vi "autogen action.vi"(8 "error in":errorcluster, 9 "user event":T1, 10 "engine configuration in":refnum<class "engine configuration.lvclass">, 11 "UI Reference configuration in":refnum<class "UI Reference configuration.lvclass">=refnum) -> (0 "error out":errorcluster, 2 "engine configuration out":refnum<class "engine configuration.lvclass">, 3 "UI Reference configuration out":refnum<class "UI Reference configuration.lvclass">)   [LabVIEW 2014, in "UI Reference editor node.lvclass"]
uses:
  UI Reference editor node.lvclass
  <vilib>/NI/Configuration Framework/Controls/EventCluster.ctl
  <vilib>/NI/Configuration Framework/NISE_CEF_TreeControl.lvlib
  <vilib>/NI/Module Execution Interface/Engine Configuration/engine configuration.lvclass
  <vilib>/NI/Configuration Framework/serializable configuration/NISE_CEF_serializable configuration.lvclass
  module/configuration/UI Reference configuration.lvclass
  <vilib>/NI/Configuration Framework/Node/UserEventRef.ctl
  <vilib>/NI/Configuration Framework/Node/NISE_CEF_Node.lvclass
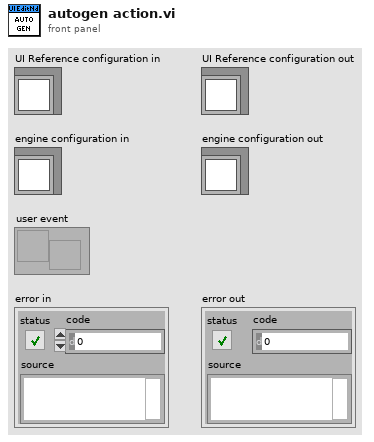
[diagram p1: front panel]
types:
  T1 = typedef "NISE_CEF_Node.lvclass/UserEventRef.ctl" = refnum<user-event>
  T2 = typedef "NISE_CEF_TreeControl.lvlib/EventCluster.ctl" = cluster{"command":string, "data":string}
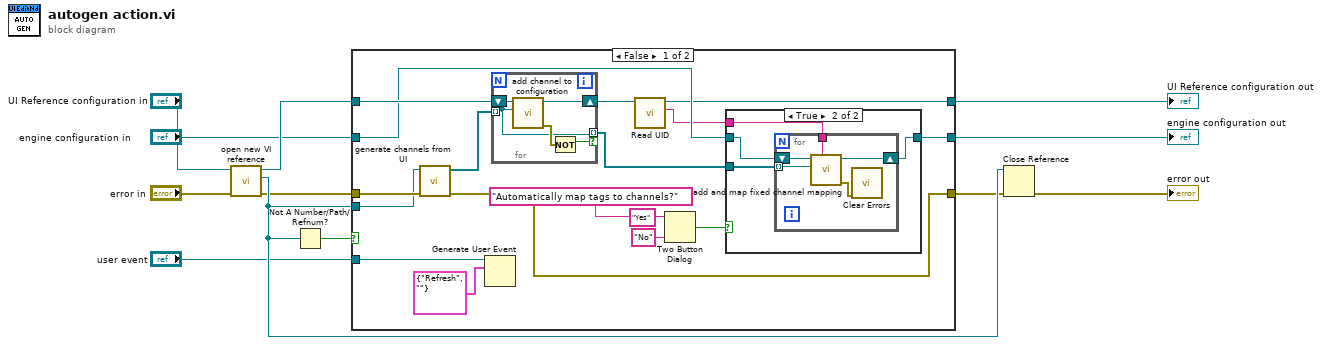
[diagram p0: block diagram]
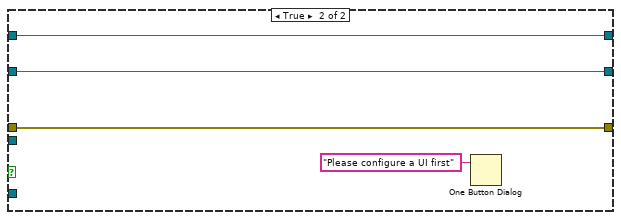
[diagram p3: hidden frame]
diagram:
  n1 = call "open new VI reference.vi"("error in"="error in", "UI Reference configuration in"="UI Reference configuration in") -> ("error out"=w7:errorcluster, "VI Refnum"=w9:refnum<vi>, "UI Reference configuration out"=w6:refnum<class "UI Reference configuration.lvclass">)  [unwired: 7 in]
  n2 = Not A Number/Path/Refnum?(number/path/refnum=w9) -> (NaN/Path/Refnum?=w1:bool)
  n3 = case shown="False" w1 {
    tunnel: w7 -> [w29 w46]
    tunnel: w6 -> [w27 w47]
    tunnel: [w20 w48] -> w11
    tunnel: "engine configuration in" -> [w21 w48]
    tunnel: [w14 w47] -> w12
    tunnel: [w18 w46] -> w3
    tunnel: w9 -> [w28 _]
    tunnel: "user event" -> [w16 _]
    frame False {
      n4 = call "generate channels from UI.vi"("error in"=w29, "VI Refnum"=w28) -> ("error out"=w18:errorcluster, "channels"=w26:refnum<class "TBM channel.lvclass">[])  [unwired: 8 in]
      n5 = Generate User Event(user event=w16, event data cluster=T2 {"command"="Refresh", "data"=""} ("event data")) -> ()  [unwired: 2 in, 2 out]
      n6 = for {
        tunnel: w26 -> [w41] mode=indexing
        shift-right: [w43] -> w22
        shift-left: w27 -> [w44]
        tunnel: [w41] -> w19 mode=indexing if=w40
        n7 = call "add channel to configuration.vi"("channel"=w41, "UI Reference configuration in"=w44) -> ("error out"=w42:errorcluster, "UI Reference configuration out"=w43:refnum<class "UI Reference configuration.lvclass">)  [unwired: 8 in]
        n8 = Not(x=w42) -> (.not. x?=w40:bool)
      }
      n9 = call <vilib>:"Read UID.vi"("configuration in"=w22) -> ("instance id"=w13:string, "configuration out"=w14:refnum<class "NISE_CEF_serializable configuration.lvclass">)  [unwired: 8 in, 1 out]
      n10 = Two Button Dialog(message="Automatically map tags to channels?", 1:"No" ("F button name (\"Cancel\")"), 2:"Yes" ("T button name (\"OK\")")) -> (T button?=w23:bool)
      n11 = case shown="True" w23 {
        tunnel: w21 -> [w30 w34]
        tunnel: [w30 w33] -> w20
        tunnel: w19 -> [_ w32]
        tunnel: w13 -> [_ w31]
        frame False {
        }
        frame True {
          n12 = for {
            shift-right: [w38] -> w33
            shift-left: w34 -> [w39]
            tunnel: w32 -> [w37] mode=indexing
            tunnel: w31 -> [w35]
            n13 = call <vilib>:"add and map fixed channel mapping.vi"("module instance"=w35, "fixed channel"=w37, "engine configuration in"=w39) -> ("error out"=w36:errorcluster, "engine configuration out"=w38:refnum<class "engine configuration.lvclass">)  [unwired: 7 in]
            n14 = call <vilib>:"Clear Errors.vi"("error in (no error)"=w36) -> ()  [unwired: 5 in, 2 out]
          }
        }
      }
    }
    frame True {
      n15 = One Button Dialog(message="Please configure a UI first") -> ()  [unwired: 1 in, 1 out]
    }
  }
  "UI Reference configuration out" <- w12
  "engine configuration out" <- w11
  n16 = Close Reference(reference=w9, error in (no error)=w3) -> (error out=→"error out":errorcluster)
